vi "experiment control.vi"() -> ()   [LabVIEW 2012] (continued)
  out "dio64:debug2":T36(array[cluster])=[{"Begin (ms)"=0.0, "Duration (ms)"=0.1720000000000006, "DIO64 Line 1"=[FALSE, FALSE, FALSE, FALSE, FALSE, FALSE, FALSE, FALSE, FALSE, FALSE, FALSE, FALSE, FALSE, FALSE, FALSE, FALSE], "DIO64 Line 2"=[FALSE, FALSE, FALSE, FALSE, FALSE, FALSE, FALSE, FALSE, FALSE, FALSE, FALSE, FALSE, FALSE, FALSE, FALSE, FALSE], "DIO64 Line 3"=[FALSE, FALSE, FALSE, FALSE, FALSE, FALSE, FALSE, FALSE, FALSE, FALSE, FALSE, FALSE, FALSE, FALSE, FALSE, FALSE], "DIO64 Line 4"=[FALSE, FALSE, FALSE, FALSE, FALSE, FALSE, FALSE, FALSE, FALSE, FALSE, FALSE, FALSE, FALSE, FALSE, FALSE, FALSE]}, {"Begin (ms)"=0.1720000000000006, "Duration (ms)"=4.020009999999999, "DIO64 Line 1"=[FALSE, FALSE, FALSE, FALSE, FALSE, FALSE, FALSE, FALSE, FALSE, FALSE, FALSE, FALSE, FALSE, TRUE, FALSE, FALSE], "DIO64 Line 2"=[FALSE, FALSE, FALSE, FALSE, FALSE, FALSE, FALSE, FALSE, FALSE, FALSE, FALSE, FALSE, FALSE, FALSE, FALSE, TRUE], "DIO64 Line 3"=[FALSE, FALSE, FALSE, FALSE, FALSE, FALSE, FALSE, FALSE, FALSE, FALSE, FALSE, FALSE, FALSE, FALSE, FALSE, FALSE], "DIO64 Line 4"=[FALSE, FALSE, FALSE, FALSE, FALSE, FALSE, FALSE, FALSE, FALSE, FALSE, FALSE, FALSE, FALSE, FALSE, FALSE, FALSE]}, {"Begin (ms)"=4.19201, "Duration (ms)"=0.010000000000001563, "DIO64 Line 1"=[FALSE, FALSE, FALSE, FALSE, FALSE, FALSE, FALSE, FALSE, FALSE, FALSE, FALSE, FALSE, FALSE, TRUE, FALSE, FALSE], "DIO64 Line 2"=[FALSE, FALSE, FALSE, FALSE, FALSE, FALSE, FALSE, FALSE, FALSE, FALSE, FALSE, FALSE, FALSE, FALSE, FALSE, TRUE], "DIO64 Line 3"=[FALSE, FALSE, FALSE, FALSE, FALSE, FALSE, FALSE, FALSE, FALSE, FALSE, FALSE, FALSE, FALSE, FALSE, FALSE, FALSE], "DIO64 Line 4"=[FALSE, FALSE, FALSE, FALSE, FALSE, FALSE, FALSE, FALSE, FALSE, FALSE, FALSE, FALSE, FALSE, FALSE, FALSE, FALSE]}, {"Begin (ms)"=4.202010000000001, "Duration (ms)"=13.97239, "DIO64 Line 1"=[FALSE, FALSE, FALSE, FALSE, FALSE, FALSE, FALSE, FALSE, FALSE, FALSE, FALSE, FALSE, FALSE, TRUE, FALSE, FALSE], "DIO64 Line 2"=[FALSE, FALSE, FALSE, FALSE, FALSE, FALSE, FALSE, FALSE, FALSE, FALSE, FALSE, FALSE, FALSE, FALSE, FALSE, TRUE], "DIO64 Line 3"=[FALSE, FALSE, FALSE, FALSE, FALSE, FALSE, FALSE, FALSE, FALSE, FALSE, FALSE, FALSE, FALSE, FALSE, FALSE, FALSE], "DIO64 Line 4"=[FALSE, FALSE, FALSE, FALSE, FALSE, FALSE, FALSE, FALSE, FALSE, FALSE, FALSE, FALSE, FALSE, FALSE, FALSE, FALSE]}, {"Begin (ms)"=18.174400000000002, "Duration (ms)"=0.00999999999999801, "DIO64 Line 1"=[FALSE, FALSE, FALSE, FALSE, FALSE, FALSE, FALSE, FALSE, FALSE, FALSE, FALSE, FALSE, FALSE, TRUE, FALSE, FALSE], "DIO64 Line 2"=[FALSE, FALSE, FALSE, FALSE, FALSE, FALSE, FALSE, FALSE, FALSE, FALSE, FALSE, FALSE, FALSE, FALSE, FALSE, TRUE], "DIO64 Line 3"=[FALSE, FALSE, FALSE, FALSE, FALSE, FALSE, FALSE, FALSE, FALSE, FALSE, FALSE, FALSE, FALSE, FALSE, FALSE, FALSE], "DIO64 Line 4"=[TRUE, FALSE, FALSE, FALSE, FALSE, FALSE, FALSE, FALSE, FALSE, FALSE, FALSE, FALSE, FALSE, FALSE, FALSE, FALSE]}, {"Begin (ms)"=18.1844, "Duration (ms)"=0.9876000000000005, "DIO64 Line 1"=[FALSE, FALSE, FALSE, FALSE, FALSE, FALSE, FALSE, FALSE, FALSE, FALSE, FALSE, FALSE, FALSE, TRUE, FALSE, FALSE], "DIO64 Line 2"=[FALSE, FALSE, FALSE, FALSE, FALSE, FALSE, FALSE, FALSE, FALSE, FALSE, FALSE, FALSE, FALSE, FALSE, FALSE, TRUE], "DIO64 Line 3"=[FALSE, FALSE, FALSE, FALSE, FALSE, FALSE, FALSE, FALSE, FALSE, FALSE, FALSE, FALSE, FALSE, FALSE, FALSE, FALSE], "DIO64 Line 4"=[FALSE, FALSE, FALSE, FALSE, FALSE, FALSE, FALSE, FALSE, FALSE, FALSE, FALSE, FALSE, FALSE, FALSE, FALSE, FALSE]}, {"Begin (ms)"=19.172, "Duration (ms)"=0.010000000000001563, "DIO64 Line 1"=[FALSE, FALSE, FALSE, FALSE, FALSE, FALSE, FALSE, FALSE, FALSE, FALSE, FALSE, FALSE, FALSE, TRUE, FALSE, FALSE], "DIO64 Line 2"=[FALSE, FALSE, FALSE, FALSE, FALSE, FALSE, FALSE, FALSE, FALSE, TRUE, FALSE, FALSE, FALSE, FALSE, FALSE, TRUE], "DIO64 Line 3"=[FALSE, FALSE, FALSE, FALSE, FALSE, FALSE, FALSE, FALSE, FALSE, FALSE, FALSE, FALSE, FALSE, FALSE, FALSE, FALSE], "DIO64 Line 4"=[FALSE, FALSE, FALSE, FALSE, FALSE, FALSE, FALSE, FALSE, FALSE, FALSE, FALSE, FALSE, FALSE, FALSE, FALSE, FALSE]}, {"Begin (ms)"=19.182000000000002, "Duration (ms)"=0.136099999999999, "DIO64 Line 1"=[FALSE, FALSE, FALSE, FALSE, FALSE, FALSE, FALSE, FALSE, FALSE, FALSE, FALSE, FALSE, FALSE, TRUE, FALSE, FALSE], "DIO64 Line 2"=[FALSE, FALSE, FALSE, FALSE, FALSE, FALSE, FALSE, FALSE, FALSE, FALSE, FALSE, FALSE, FALSE, FALSE, FALSE, TRUE], "DIO64 Line 3"=[FALSE, FALSE, FALSE, FALSE, FALSE, FALSE, FALSE, FALSE, FALSE, FALSE, FALSE, FALSE, FALSE, FALSE, FALSE, FALSE], "DIO64 Line 4"=[FALSE, FALSE, FALSE, FALSE, FALSE, FALSE, FALSE, FALSE, FALSE, FALSE, FALSE, FALSE, FALSE, FALSE, FALSE, FALSE]}, {"Begin (ms)"=19.3181, "Duration (ms)"=0.010000000000001563, "DIO64 Line 1"=[FALSE, FALSE, FALSE, TRUE, FALSE, FALSE, FALSE, FALSE, FALSE, FALSE, FALSE, FALSE, FALSE, TRUE, TRUE, FALSE], "DIO64 Line 2"=[FALSE, FALSE, FALSE, FALSE, FALSE, FALSE, FALSE, FALSE, FALSE, FALSE, FALSE, FALSE, FALSE, FALSE, FALSE, TRUE], "DIO64 Line 3"=[FALSE, FALSE, FALSE, FALSE, FALSE, FALSE, FALSE, FALSE, FALSE, FALSE, FALSE, FALSE, FALSE, FALSE, FALSE, FALSE], "DIO64 Line 4"=[FALSE, FALSE, FALSE, FALSE, FALSE, FALSE, FALSE, FALSE, FALSE, FALSE, FALSE, FALSE, FALSE, FALSE, FALSE, FALSE]}, {"Begin (ms)"=19.328100000000003, "Duration (ms)"=0.054999999999999716, "DIO64 Line 1"=[FALSE, FALSE, FALSE, FALSE, FALSE, FALSE, FALSE, FALSE, FALSE, FALSE, FALSE, FALSE, FALSE, TRUE, TRUE, FALSE], "DIO64 Line 2"=[FALSE, FALSE, FALSE, FALSE, FALSE, FALSE, FALSE, FALSE, FALSE, FALSE, FALSE, FALSE, FALSE, FALSE, FALSE, TRUE], "DIO64 Line 3"=[FALSE, FALSE, FALSE, FALSE, FALSE, FALSE, FALSE, FALSE, FALSE, FALSE, FALSE, FALSE, FALSE, FALSE, FALSE, FALSE], "DIO64 Line 4"=[FALSE, FALSE, FALSE, FALSE, FALSE, FALSE, FALSE, FALSE, FALSE, FALSE, FALSE, FALSE, FALSE, FALSE, FALSE, FALSE]}, {"Begin (ms)"=19.383100000000002, "Duration (ms)"=0.06009999999999849, "DIO64 Line 1"=[FALSE, FALSE, FALSE, FALSE, FALSE, FALSE, FALSE, FALSE, FALSE, FALSE, FALSE, FALSE, FALSE, TRUE, FALSE, FALSE], "DIO64 Line 2"=[FALSE, FALSE, FALSE, FALSE, FALSE, FALSE, FALSE, FALSE, FALSE, FALSE, FALSE, FALSE, FALSE, FALSE, FALSE, TRUE], "DIO64 Line 3"=[FALSE, FALSE, FALSE, FALSE, FALSE, FALSE, FALSE, FALSE, FALSE, FALSE, FALSE, FALSE, FALSE, FALSE, FALSE, FALSE], "DIO64 Line 4"=[FALSE, FALSE, FALSE, FALSE, FALSE, FALSE, FALSE, FALSE, FALSE, FALSE, FALSE, FALSE, FALSE, FALSE, FALSE, FALSE]}, {"Begin (ms)"=19.4432, "Duration (ms)"=0.010000000000001563, "DIO64 Line 1"=[FALSE, FALSE, FALSE, FALSE, TRUE, FALSE, FALSE, FALSE, FALSE, FALSE, FALSE, FALSE, FALSE, TRUE, FALSE, FALSE], "DIO64 Line 2"=[FALSE, FALSE, FALSE, FALSE, FALSE, FALSE, FALSE, FALSE, FALSE, FALSE, FALSE, FALSE, FALSE, FALSE, FALSE, TRUE], "DIO64 Line 3"=[FALSE, FALSE, FALSE, FALSE, FALSE, FALSE, FALSE, FALSE, FALSE, FALSE, FALSE, FALSE, FALSE, FALSE, FALSE, FALSE], "DIO64 Line 4"=[FALSE, FALSE, FALSE, FALSE, FALSE, FALSE, FALSE, FALSE, FALSE, FALSE, FALSE, FALSE, FALSE, FALSE, FALSE, FALSE]}, {"Begin (ms)"=19.453200000000002, "Duration (ms)"=0.6777999999999977, "DIO64 Line 1"=[FALSE, FALSE, FALSE, FALSE, FALSE, FALSE, FALSE, FALSE, FALSE, FALSE, FALSE, FALSE, FALSE, TRUE, FALSE, FALSE], "DIO64 Line 2"=[FALSE, FALSE, FALSE, FALSE, FALSE, FALSE, FALSE, FALSE, FALSE, FALSE, FALSE, FALSE, FALSE, FALSE, FALSE, TRUE], "DIO64 Line 3"=[FALSE, FALSE, FALSE, FALSE, FALSE, FALSE, FALSE, FALSE, FALSE, FALSE, FALSE, FALSE, FALSE, FALSE, FALSE, FALSE], "DIO64 Line 4"=[FALSE, FALSE, FALSE, FALSE, FALSE, FALSE, FALSE, FALSE, FALSE, FALSE, FALSE, FALSE, FALSE, FALSE, FALSE, FALSE]}, {"Begin (ms)"=20.131, "Duration (ms)"=0.03999999999999915, "DIO64 Line 1"=[FALSE, FALSE, FALSE, FALSE, FALSE, FALSE, FALSE, FALSE, FALSE, TRUE, TRUE, FALSE, FALSE, TRUE, FALSE, FALSE], "DIO64 Line 2"=[FALSE, FALSE, FALSE, FALSE, FALSE, FALSE, FALSE, FALSE, FALSE, FALSE, FALSE, FALSE, FALSE, FALSE, FALSE, TRUE], "DIO64 Line 3"=[FALSE, FALSE, FALSE, FALSE, FALSE, FALSE, FALSE, FALSE, FALSE, FALSE, FALSE, FALSE, FALSE, FALSE, FALSE, FALSE], "DIO64 Line 4"=[FALSE, FALSE, FALSE, FALSE, FALSE, FALSE, FALSE, FALSE, FALSE, FALSE, FALSE, FALSE, FALSE, FALSE, FALSE, FALSE]}, {"Begin (ms)"=20.171, "Duration (ms)"=0.0010000000000012221, "DIO64 Line 1"=[FALSE, FALSE, FALSE, FALSE, FALSE, FALSE, FALSE, FALSE, FALSE, TRUE, FALSE, FALSE, FALSE, TRUE, FALSE, FALSE], "DIO64 Line 2"=[FALSE, FALSE, FALSE, FALSE, FALSE, FALSE, FALSE, FALSE, FALSE, FALSE, FALSE, FALSE, FALSE, FALSE, FALSE, TRUE], "DIO64 Line 3"=[FALSE, FALSE, FALSE, FALSE, FALSE, FALSE, FALSE, FALSE, FALSE, FALSE, FALSE, FALSE, FALSE, FALSE, FALSE, FALSE], "DIO64 Line 4"=[FALSE, FALSE, FALSE, FALSE, FALSE, FALSE, FALSE, FALSE, FALSE, FALSE, FALSE, FALSE, FALSE, FALSE, FALSE, FALSE]}, {"Begin (ms)"=20.172, "Duration (ms)"=2.0, "DIO64 Line 1"=[FALSE, FALSE, FALSE, FALSE, FALSE, FALSE, TRUE, FALSE, FALSE, FALSE, FALSE, FALSE, FALSE, TRUE, FALSE, FALSE], "DIO64 Line 2"=[FALSE, FALSE, FALSE, FALSE, TRUE, FALSE, FALSE, FALSE, FALSE, FALSE, FALSE, FALSE, FALSE, TRUE, FALSE, TRUE], "DIO64 Line 3"=[FALSE, FALSE, FALSE, TRUE, FALSE, FALSE, FALSE, FALSE, FALSE, FALSE, FALSE, FALSE, FALSE, FALSE, FALSE, FALSE], "DIO64 Line 4"=[FALSE, FALSE, FALSE, FALSE, FALSE, FALSE, FALSE, FALSE, FALSE, FALSE, FALSE, FALSE, FALSE, FALSE, FALSE, TRUE]}, {"Begin (ms)"=22.172, "Duration (ms)"=0.004999999999999005, "DIO64 Line 1"=[FALSE, FALSE, FALSE, FALSE, FALSE, FALSE, FALSE, FALSE, FALSE, TRUE, FALSE, FALSE, FALSE, TRUE, FALSE, FALSE], "DIO64 Line 2"=[FALSE, FALSE, FALSE, FALSE, FALSE, FALSE, FALSE, FALSE, FALSE, FALSE, FALSE, TRUE, FALSE, FALSE, FALSE, TRUE], "DIO64 Line 3"=[FALSE, FALSE, FALSE, FALSE, FALSE, FALSE, FALSE, FALSE, FALSE, FALSE, FALSE, FALSE, FALSE, FALSE, FALSE, FALSE], "DIO64 Line 4"=[FALSE, FALSE, FALSE, FALSE, FALSE, FALSE, FALSE, FALSE, FALSE, FALSE, FALSE, FALSE, FALSE, FALSE, FALSE, FALSE]}, {"Begin (ms)"=22.177, "Duration (ms)"=0.005000000000002558, "DIO64 Line 1"=[FALSE, FALSE, FALSE, FALSE, FALSE, FALSE, FALSE, FALSE, FALSE, TRUE, TRUE, FALSE, FALSE, TRUE, FALSE, FALSE], "DIO64 Line 2"=[FALSE, FALSE, FALSE, FALSE, FALSE, FALSE, FALSE, FALSE, FALSE, FALSE, FALSE, TRUE, FALSE, FALSE, FALSE, TRUE], "DIO64 Line 3"=[FALSE, FALSE, FALSE, FALSE, FALSE, FALSE, FALSE, FALSE, FALSE, FALSE, FALSE, FALSE, FALSE, FALSE, FALSE, FALSE], "DIO64 Line 4"=[FALSE, FALSE, FALSE, FALSE, FALSE, FALSE, FALSE, FALSE, FALSE, FALSE, FALSE, FALSE, FALSE, FALSE, FALSE, FALSE]}, {"Begin (ms)"=22.182000000000002, "Duration (ms)"=0.004999999999999005, "DIO64 Line 1"=[FALSE, FALSE, FALSE, FALSE, FALSE, FALSE, FALSE, FALSE, FALSE, TRUE, TRUE, FALSE, FALSE, TRUE, FALSE, FALSE], "DIO64 Line 2"=[FALSE, FALSE, FALSE, FALSE, FALSE, FALSE, FALSE, FALSE, FALSE, FALSE, FALSE, FALSE, FALSE, FALSE, FALSE, TRUE], "DIO64 Line 3"=[FALSE, FALSE, FALSE, FALSE, FALSE, FALSE, FALSE, FALSE, FALSE, FALSE, FALSE, FALSE, FALSE, FALSE, FALSE, FALSE], "DIO64 Line 4"=[FALSE, FALSE, FALSE, FALSE, FALSE, FALSE, FALSE, FALSE, FALSE, FALSE, FALSE, FALSE, FALSE, FALSE, FALSE, FALSE]}, {"Begin (ms)"=22.187, "Duration (ms)"=0.005009999999998627, "DIO64 Line 1"=[FALSE, FALSE, FALSE, FALSE, FALSE, FALSE, FALSE, TRUE, FALSE, TRUE, TRUE, FALSE, FALSE, TRUE, FALSE, FALSE], "DIO64 Line 2"=[FALSE, FALSE, FALSE, FALSE, FALSE, FALSE, FALSE, FALSE, FALSE, FALSE, FALSE, FALSE, FALSE, FALSE, FALSE, TRUE], "DIO64 Line 3"=[FALSE, FALSE, FALSE, FALSE, FALSE, FALSE, FALSE, FALSE, FALSE, FALSE, FALSE, FALSE, FALSE, FALSE, FALSE, FALSE], "DIO64 Line 4"=[FALSE, TRUE, FALSE, FALSE, FALSE, FALSE, FALSE, FALSE, FALSE, FALSE, FALSE, FALSE, FALSE, FALSE, FALSE, FALSE]}, {"Begin (ms)"=22.19201, "Duration (ms)"=0.004989999999999384, "DIO64 Line 1"=[FALSE, FALSE, FALSE, FALSE, FALSE, FALSE, FALSE, TRUE, FALSE, TRUE, TRUE, FALSE, FALSE, TRUE, FALSE, FALSE], "DIO64 Line 2"=[FALSE, FALSE, FALSE, FALSE, FALSE, FALSE, FALSE, FALSE, FALSE, FALSE, FALSE, FALSE, FALSE, FALSE, FALSE, TRUE], "DIO64 Line 3"=[FALSE, FALSE, FALSE, FALSE, FALSE, FALSE, FALSE, FALSE, FALSE, FALSE, FALSE, FALSE, FALSE, FALSE, FALSE, FALSE], "DIO64 Line 4"=[FALSE, TRUE, FALSE, FALSE, FALSE, FALSE, FALSE, FALSE, FALSE, FALSE, FALSE, FALSE, FALSE, FALSE, FALSE, FALSE]}, {"Begin (ms)"=22.197, "Duration (ms)"=0.005010000000002179, "DIO64 Line 1"=[FALSE, FALSE, FALSE, FALSE, FALSE, FALSE, FALSE, FALSE, FALSE, TRUE, TRUE, FALSE, FALSE, TRUE, FALSE, FALSE], "DIO64 Line 2"=[FALSE, FALSE, FALSE, FALSE, FALSE, FALSE, FALSE, FALSE, FALSE, FALSE, FALSE, FALSE, FALSE, FALSE, FALSE, TRUE], "DIO64 Line 3"=[FALSE, FALSE, FALSE, FALSE, FALSE, FALSE, FALSE, FALSE, FALSE, FALSE, FALSE, FALSE, FALSE, FALSE, FALSE, FALSE], "DIO64 Line 4"=[FALSE, FALSE, FALSE, FALSE, FALSE, FALSE, FALSE, FALSE, FALSE, FALSE, FALSE, FALSE, FALSE, FALSE, FALSE, FALSE]}, {"Begin (ms)"=22.20201, "Duration (ms)"=9.974989999999998, "DIO64 Line 1"=[FALSE, FALSE, FALSE, FALSE, FALSE, FALSE, FALSE, FALSE, FALSE, TRUE, TRUE, FALSE, FALSE, TRUE, FALSE, FALSE], "DIO64 Line 2"=[FALSE, FALSE, FALSE, FALSE, FALSE, FALSE, FALSE, FALSE, FALSE, FALSE, FALSE, FALSE, FALSE, FALSE, FALSE, TRUE], "DIO64 Line 3"=[FALSE, FALSE, FALSE, FALSE, FALSE, FALSE, FALSE, FALSE, FALSE, FALSE, FALSE, FALSE, FALSE, FALSE, FALSE, FALSE], "DIO64 Line 4"=[FALSE, FALSE, FALSE, FALSE, FALSE, FALSE, FALSE, FALSE, FALSE, FALSE, FALSE, FALSE, FALSE, FALSE, FALSE, FALSE]}, {"Begin (ms)"=32.177, "Duration (ms)"=67.995, "DIO64 Line 1"=[FALSE, FALSE, FALSE, FALSE, FALSE, FALSE, FALSE, FALSE, FALSE, FALSE, FALSE, FALSE, FALSE, TRUE, FALSE, FALSE], "DIO64 Line 2"=[FALSE, FALSE, FALSE, FALSE, FALSE, FALSE, FALSE, FALSE, FALSE, FALSE, FALSE, FALSE, FALSE, FALSE, FALSE, TRUE], "DIO64 Line 3"=[FALSE, FALSE, FALSE, FALSE, FALSE, FALSE, FALSE, FALSE, FALSE, FALSE, FALSE, FALSE, FALSE, FALSE, FALSE, FALSE], "DIO64 Line 4"=[FALSE, FALSE, FALSE, FALSE, FALSE, FALSE, FALSE, FALSE, FALSE, FALSE, FALSE, FALSE, FALSE, FALSE, FALSE, FALSE]}, {"Begin (ms)"=100.172, "Duration (ms)"=99.828, "DIO64 Line 1"=[FALSE, FALSE, FALSE, FALSE, FALSE, FALSE, FALSE, FALSE, FALSE, FALSE, FALSE, FALSE, FALSE, FALSE, FALSE, FALSE], "DIO64 Line 2"=[FALSE, FALSE, FALSE, FALSE, FALSE, FALSE, FALSE, FALSE, FALSE, FALSE, FALSE, FALSE, FALSE, FALSE, FALSE, FALSE], "DIO64 Line 3"=[FALSE, FALSE, FALSE, FALSE, FALSE, FALSE, FALSE, FALSE, FALSE, FALSE, FALSE, FALSE, FALSE, FALSE, FALSE, FALSE], "DIO64 Line 4"=[FALSE, FALSE, FALSE, FALSE, FALSE, FALSE, FALSE, FALSE, FALSE, FALSE, FALSE, FALSE, FALSE, FALSE, FALSE, FALSE]}] caption="DIO64 Debug Timing"
  out "dio64:debug1":T37(array[cluster])=[{"Task"="T0", "begin time"=0.0, "end time"=0.0, "Chops"=[]}, {"Task"="Bertha UV Shutter", "begin time"=0.1720000000000006, "end time"=100.172, "Chops"=[FALSE, FALSE, FALSE, FALSE, FALSE, FALSE, FALSE, FALSE, FALSE, FALSE, FALSE, FALSE]}, {"Task"="Jessica Shutter", "begin time"=0.1720000000000006, "end time"=100.172, "Chops"=[FALSE, FALSE, FALSE, FALSE, FALSE, FALSE, FALSE, FALSE, FALSE, FALSE, FALSE, FALSE]}, {"Task"="Framegrabber Trigger", "begin time"=4.19201, "end time"=4.202010000000001, "Chops"=[TRUE, TRUE, TRUE, TRUE, TRUE, TRUE, FALSE, FALSE, FALSE, FALSE, FALSE, FALSE]}, {"Task"="IOUpdate", "begin time"=18.174400000000002, "end time"=18.1844, "Chops"=[FALSE, FALSE, FALSE, FALSE, FALSE, FALSE, FALSE, FALSE, FALSE, FALSE, FALSE, FALSE]}, {"Task"="Trigger DAC", "begin time"=19.172, "end time"=19.182000000000002, "Chops"=[FALSE, FALSE, FALSE, FALSE, FALSE, FALSE, FALSE, FALSE, FALSE, FALSE, FALSE, FALSE]}, {"Task"="Abby Flashlamp", "begin time"=19.3181, "end time"=19.328100000000003, "Chops"=[FALSE, FALSE, FALSE, FALSE, FALSE, FALSE, FALSE, FALSE, FALSE, FALSE, FALSE, FALSE]}, {"Task"="Gas Pulse", "begin time"=19.3181, "end time"=19.383100000000002, "Chops"=[FALSE, FALSE, FALSE, FALSE, FALSE, FALSE, FALSE, FALSE, FALSE, FALSE, FALSE, FALSE]}, {"Task"="Abby Q-switch", "begin time"=19.4432, "end time"=19.453200000000002, "Chops"=[FALSE, FALSE, FALSE, FALSE, FALSE, FALSE, FALSE, FALSE, FALSE, FALSE, FALSE, FALSE]}, {"Task"="Zero DAC", "begin time"=20.131, "end time"=20.171, "Chops"=[FALSE, FALSE, FALSE, FALSE, FALSE, FALSE, FALSE, FALSE, FALSE, FALSE, FALSE, FALSE]}, {"Task"="Stop Ions", "begin time"=20.171, "end time"=20.172, "Chops"=[FALSE, FALSE, FALSE, FALSE, FALSE, FALSE, FALSE, FALSE, FALSE, FALSE, FALSE, FALSE]}, {"Task"="Trap", "begin time"=20.172, "end time"=22.172, "Chops"=[FALSE, FALSE, FALSE, FALSE, FALSE, FALSE, FALSE, FALSE, FALSE, FALSE, FALSE, FALSE]}, {"Task"="Kick to MCP", "begin time"=22.172, "end time"=22.177, "Chops"=[FALSE, FALSE, FALSE, FALSE, FALSE, FALSE, FALSE, FALSE, FALSE, FALSE, FALSE, FALSE]}, {"Task"="Scope trigger 2", "begin time"=22.172, "end time"=22.182000000000002, "Chops"=[TRUE, TRUE, TRUE, FALSE, FALSE, FALSE, FALSE, FALSE, FALSE, FALSE, FALSE, FALSE]}, {"Task"="Zero DAC", "begin time"=22.177, "end time"=32.177, "Chops"=[FALSE, FALSE, FALSE, FALSE, FALSE, FALSE, FALSE, FALSE, FALSE, FALSE, FALSE, FALSE]}, {"Task"="Trigger Scope", "begin time"=22.187, "end time"=22.197, "Chops"=[FALSE, FALSE, FALSE, FALSE, FALSE, FALSE, TRUE, FALSE, FALSE, FALSE, FALSE, FALSE]}, {"Task"="Img MCP Trigger", "begin time"=22.19201, "end time"=22.20201, "Chops"=[TRUE, TRUE, TRUE, TRUE, TRUE, TRUE, FALSE, FALSE, FALSE, FALSE, FALSE, FALSE]}] caption="DIO64 Debug Timing" {"end time" format="%#_8g"; "begin time" format="%#_8g"}
  out "toptica:task:skip":refnum<k21>
  out "stella:task:skip":refnum<k21>
  out "TDS5034B Data":cluster{"Y":dbl[], "t0":dbl, "dt":dbl}[](array[cluster])=[{"Y"=array[2500 elements], "t0"=3.7485e-09, "dt"=4e-09}]
  out "documentation":string[](array[string])=["Initialize the shift-register data, here.\n(data names are defined by what you wire into the bundle function)", "Cleanup any data and references, here.\n(this is called automatically, by the Macro: Exit)", "Initialize the User Interface, here.\n(this is called automatically, by the Macro: Init)", "Set and Unset Cursor Busy.\n(Usage: \"UI: Cursor Set >> Busy|Idle\")", "Argument", "Gets the program states from the main loop case selector\n(Usage: \"UI: Get Case Strings\")", "Gets program documentation from main loop case selector\n(Usage: \"UI: Get Case Documentation\")", "Updates DIO64 control with string from DIO64 Tasks\n(Usage: \"call after any modification to DIO64 Tasks\")", "Updates DIO64 control with string from DIO64 Tasks\n(Usage: \"call after any modification to DIO64 Tasks\")", "Updates DIO64 control with string from DIO64 Tasks\n(Usage: \"call after any modification to DIO64 Tasks\")", "Initialization Macro\n(This is called once, when the VI starts. It calls a number of other program states.)", "Exit Macro\n(This is called once, when the VI exits)", "Delays for some number of milliseconds\n(Usage: delay >>  TIME)", "Prints a message to the labview stdout control\n(Usage: stdout >> TEXT)", "Clears the queue\n(Usage: abort)", "Runs the test sequence\n(Usage: Test)", "Pauses the state machine\n(swaps out the queue to memory)", "Pauses the state machine\n(swaps out the queue to memory)", "Pauses the state machine\n(swaps out the queue to memory)", "Pauses the state machine\n(swaps out the queue to memory)", "Initialize the DIO64", "Parses the DIO64\n(Usage: DIO64: Prepare >> CHOP)", "Updates the DIO64 Timing Graph\n(Usage: call whenever the DIO64 changes)", "Runs the DIO64\n(Usage: DIO64: Run )\n(Usage: DIO64: Run >> Chop,CHOP to run CHOP a number of times in the frame control)\n(Usage: DIO64: Run >> Repeat,N, to run the prepared sequence N times)", "DIO64: Override\n(Usage: DIO64: Override >> CHANNEL, to run a channel like A0 or C6)", "Closes the DIO64\n(Usage: DIO64: Close)", "Initalize the Scope\n(Usage: Scope: Initialize >> SCOPE, where SCOPE can be DPO)", "Updates Scope Settings\n(Usage: Scope: Settings >> SCOPE, where SCOPE can be DPO)", "Reads a frame from the Scope\n(Usage: Scope: Read >> SCOPE, where SCOPE can be DPO)", "Close the Scope\n(Usage: Scope: Close >> SCOPE, where SCOPE can be DPO)"] caption="Documentation"
  in  "Coils AO Task:skip":refnum<k21>
  in  "Coils DO Task:skip":refnum<k21>
  out "Waveform Chart":waveform(dbl)[](graph)=[{"t0"=timestamp(0 s since 1904-01-01), "dt"=4e-09, "Y"=array[2500 elements]}]
  in  "stdin":string="Magnetometer: Close"
  # "Task Name"
  # "Start (ms)"
  # "Edge"
  # "Reference"
  # "End (ms)"
  # "Edge"
  # "Reference"
  # "Time (ms)"
  # "A0"
  # "A1"
  # "A2"
  # "A3"
  # "A4"
  # "A5"
  # "A6"
  # "Time (ms)"
  # "A0"
  # "A1"
  # "A2"
  # "A3"
  # "A4"
  # "A5"
  # "A6"
  # "A7"
  # "0"
  # "1"
  # "2"
  # "3"
  # "4"
  # "5"
  # "6"
  # "7"
  # "8"
  # "9"
  # "10"
  # "11"
  # "AO1"
  # "DO1 - Abby intlk 1"
  # "DI1"
  # "DO2 - Abby intlk 2"
  # "DI2"
  # "AO2"
  # "DO3 - Bertha WP flip"
  # "DI3"
  # "AI1"
  # "DO4 - Depletion flip"
  # "DI4"
  # "AI2"
  # "DO5"
  # "DI5"
  # "DO6"
  # "DO7"
  # "DO8"
  # "V"
  # "kHz"
  # "mVpp"
  # "deg"
  # "Freq (Hz)"
  # "Phase (deg)"
  # "Duty Cyc. (%)"
  # "Trig."
  # "1"
  # "2"
  # "(A)"
  # "(A)"
  # "(A)"
  # "(V)"
  # "(A)"
  # "(A)"
  # "(A)"
  # "(V)"
  # "(A)"
  # "(A)"
  # "(A)"
  # "(V)"
  # "(A)"
  # "(A)"
  # "(A)"
  # "(V)"
  # "nm"
  # "cm-1"
  # "Stella"
  # "Toptica"
  # "Frequency (kHz)"
  # "Phase"
  # "Amplitude"
  # "1"
  # "2"
  # "3"
  # "4"
  # "5"
  # "6"
  # "x 20 us"
  # "For Profile Pin\nAmplitude Ramps"
  # "Start"
  # "End"
  # "Ramp Time (us)"
  # "R0"
  # "R1"
  # "R2"
  # "R3"
  # "R4"
  # "R5"
  # "R6"
  # "R7"
  # "R8"
  # "R9"
  # "Hz"
  # "Hz"
  # "Hz"
  # "V"
  # "V"
  # "V"
  # "V"
  # "0"
  # "1"
  # "2"
  # "3"
  # "0"
  # "1"
  # "2"
  # "3"
  # "4"
  # "5"
  # "6"
  # "7"
  # "8"
  # "9"
  # "10"
  # "A00"
  # "A01"
  # "A02"
  # "A03"
  # "A04"
  # "A05"
  # "A06"
  # "A07"
  # "A08"
  # "A09"
  # "A10"
  # "A11"
  # "A12"
  # "A13"
  # "A14"
  # "A15"
  # "B00"
  # "B01"
  # "B02"
  # "B03"
  # "B04"
  # "B05"
  # "B06"
  # "B07"
  # "B08"
  # "B09"
  # "B10"
  # "B11"
  # "B12"
  # "B13"
  # "B14"
  # "B15"
  # "C00"
  # "C01"
  # "C02"
  # "C03"
  # "C04"
  # "C05"
  # "C06"
  # "C07"
  # "C08"
  # "C09"
  # "C10"
  # "C11"
  # "C12"
  # "C13"
  # "C14"
  # "C15"
  # "D00"
  # "D01"
  # "D02"
  # "D03"
  # "D04"
  # "D05"
  # "D06"
  # "D07"
  # "D08"
  # "D09"
  # "D10"
  # "D11"
  # "D12"
  # "D13"
  # "D14"
  # "D15"
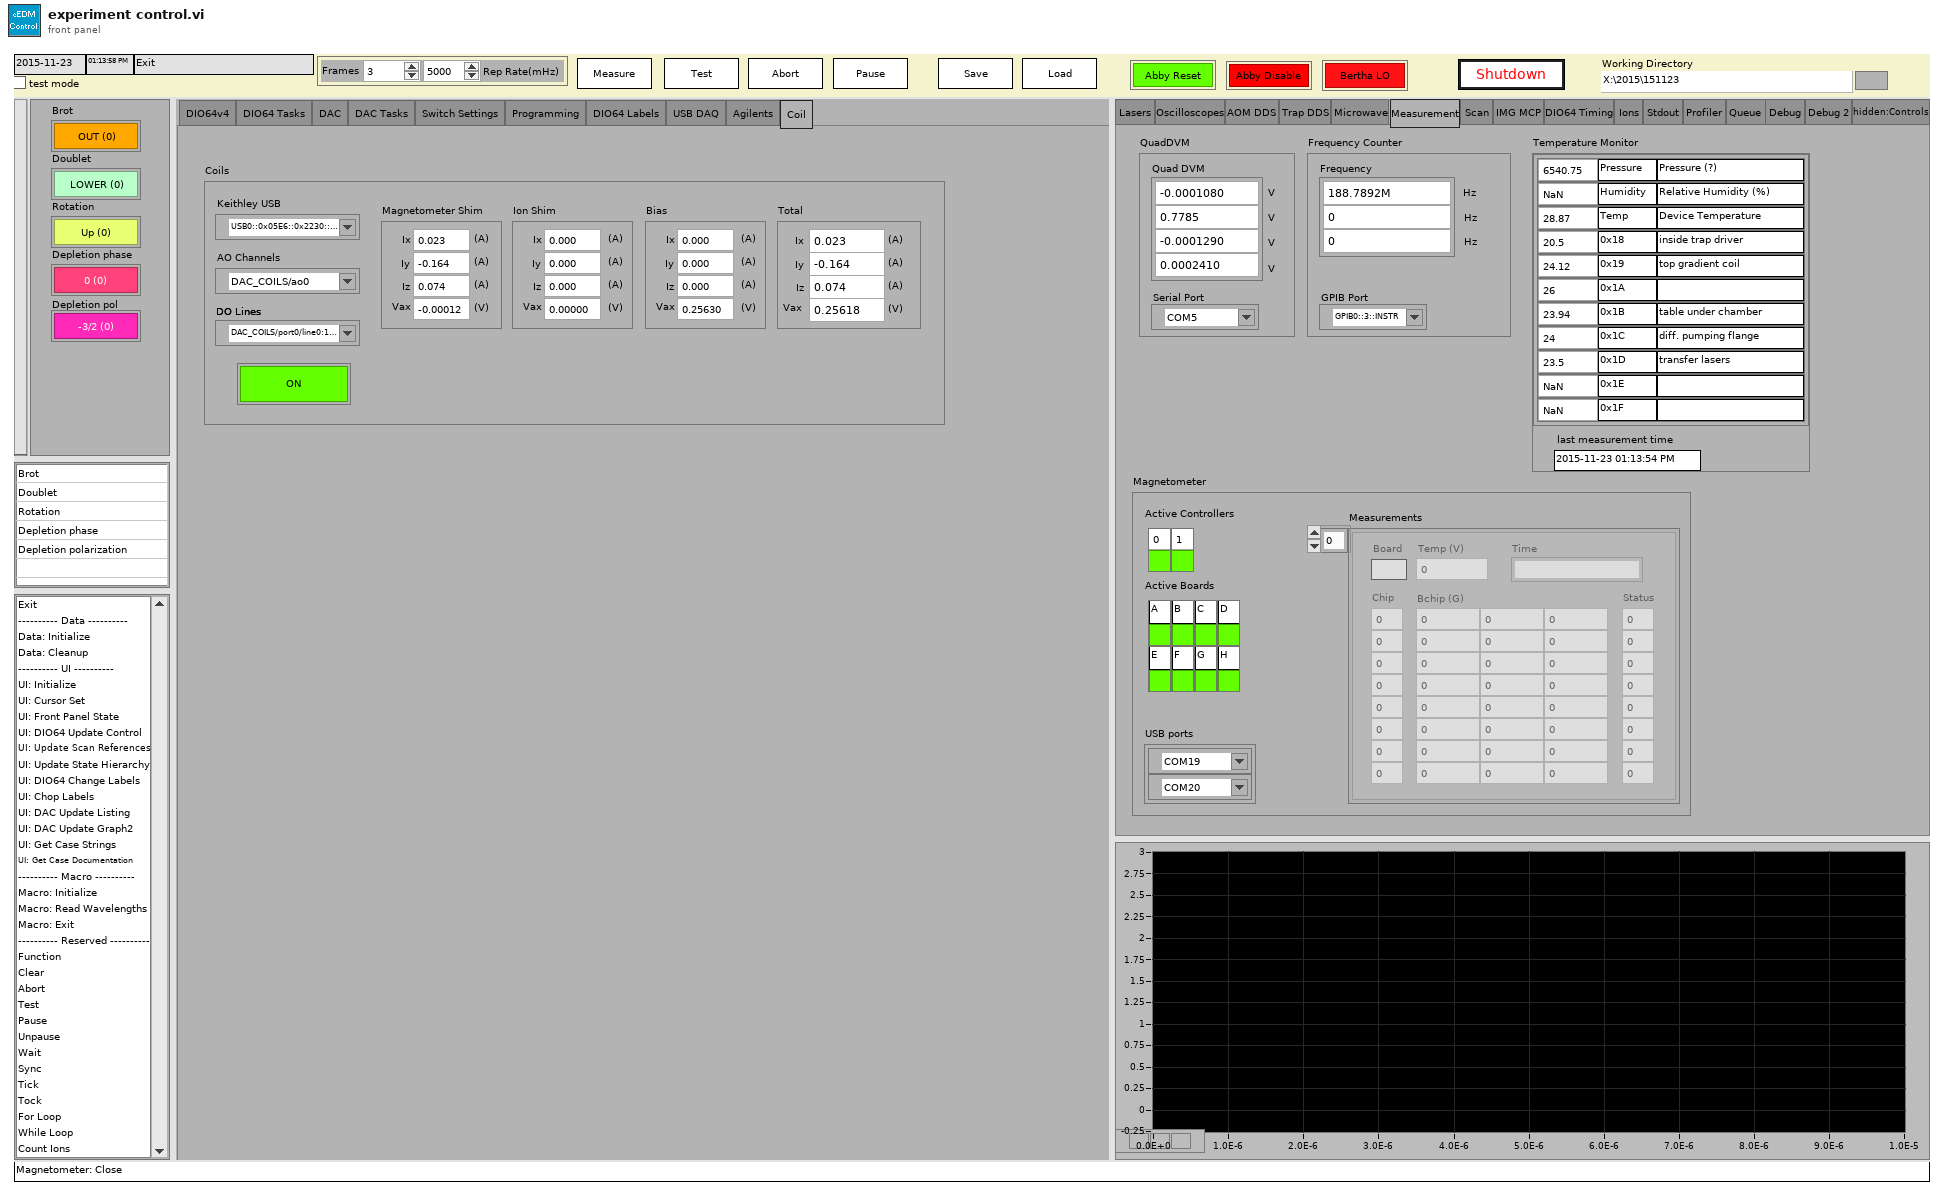
[diagram p1: front panel]
types:
  T1 = cluster{"Brot":bool, "Doublet":bool, "Rotation":bool, "Depletion phase":bool, "Depletion pol":bool}
  T2 = enum32{"DIO64v4", "DIO64 Tasks", "DAC", "DAC Tasks", "Switch Settings", "Programming", "DIO64 Labels", "USB DAQ", "Agilents", "Coil"}
  T3 = cluster{"Task":string, "begin time":dbl, "begin edge":bool, "begin reference":string, "end time":dbl, "end edge":bool, "end reference":string, "Chops":bool[]}[]
  T4 = cluster{"Name":string, "DIO64 Line 1":bool[], "DIO64 Line 2":bool[], "DIO64 Line 3":bool[], "DIO64 Line 4":bool[]}[]
  T5 = cluster{"Channel 1":picture[], "Channel 2":picture[], "Channel 3":picture[], "Channel 4":picture[]}
  T6 = cluster{"Task":string, "Reference":string, "Begin":dbl, "Chops 2":bool[]}[]
  T7 = cluster{"loaded":bool, "output 1":refnum<k21>, "clock 1":refnum<k21>, "output 2":refnum<k21>, "clock 2":refnum<k21>}
  T8 = cluster{"Name":string, "DAC":cluster{"Time":dbl, "Voltage":dbl[]}[]}[]
  T9 = cluster{"Brot":cluster{"in":dbl, "out":dbl}, "Doublet":cluster{"upper":dbl, "lower":dbl, "DurationUpper":dbl, "DurationLower":dbl, "Upper T":dbl, "Lower T":dbl}, "Rotation":cluster{"Down":cluster{"Frequency":dbl, "Phase":dbl, "Amplitude":dbl}[], "Up":cluster{"Frequency":dbl, "Phase":dbl, "Amplitude":dbl}[]}, "Depletion phase":cluster{"0 phase":dbl, "pi phase":dbl}}
  T10 = cluster{"Channel":string, "Name":string, "plot":bool}[][]
  T11 = cluster{"Digital Out":bool[], "Digital In":bool[], "Analog Out":u8[], "Analog In":u8[]}
  T12 = cluster{"Chillax":refnum<visa-resource-name>, "Output":bool, "Chillax Voltage":dbl, "Unchillax":refnum<visa-resource-name>}
  T13 = cluster{"USB":refnum<visa-resource-name>, "Amplitude":dbl, "Frequency":dbl, "Phase":dbl, "Upload":bool, "Output":bool}
  T14 = cluster{"USB":refnum<visa-resource-name>, "Upload":bool, "Output":bool, "Channels":cluster{"Frequency":dbl, "Phase":dbl, "Duty Cycle":dbl, "Trigger":bool}[], "Output Select":bool, "Amplitude":dbl, "Offset":dbl}
  T15 = cluster{"AO Channels":tag, "DO Lines":tag, "Keithley USB":refnum<visa-resource-name>, "Current Toggle":bool, "Magnetometer Shim":cluster{"x":dbl, "y":dbl, "z":dbl, "axgrad":dbl}, "Ion Shim":cluster{"x":dbl, "y":dbl, "z":dbl, "axgrad":dbl}, "Bias":cluster{"x":dbl, "y":dbl, "z":dbl, "axgrad":dbl}, "Total":cluster{"x":dbl, "y":dbl, "z":dbl, "axgrad":dbl}}
  T16 = enum32{"Lasers", "Oscilloscopes", "AOM DDS", "Trap DDS", "Microwave", "Measurement", "Scan", "IMG MCP", "DIO64 Timing", "Ions", "Stdout", "Profiler", "Queue", "Debug", "Debug 2", "hidden:Controls"}
  T17 = typedef "Laser.ctl" = cluster{"wavelength":dbl, "locked":bool, "lock tolerance":dbl, "setpoint":dbl, "scan start":dbl, "scan end":dbl, "progress":u8, "scan step":dbl, "scan":bool, "wavelengths":dbl[]}
  T18 = cluster{"wavelength":dbl, "scan start":dbl, "scan end":dbl, "progress":u8, "scan step":dbl, "scan":bool, "setpoint":dbl, "wavelengths":dbl[], "Channel":tag, "wavelength 2":dbl}
  T19 = cluster{"wavelength":dbl, "locked":bool, "scan start":dbl, "scan end":dbl, "progress":u8, "scan step":dbl, "scan":bool, "AI Channel":tag}
  T20 = cluster{"wavelength":dbl, "locked":bool, "lock tolerance":dbl, "setpoint":dbl, "scan start":dbl, "scan end":dbl, "progress":u8, "scan step":dbl, "scan":bool, "AI Channel":tag}
  T21 = cluster{"wavelength":dbl, "locked":bool, "DIO64":string, "scan start":dbl, "scan end":dbl, "progress":u8, "scan step":dbl, "scan":bool, "setpoint":dbl}
  T22 = cluster{"wavelength":dbl, "locked":bool, "DIO64":string, "scan start":dbl, "scan end":dbl, "progress":u8, "scan step":dbl, "scan":bool, "setpoint":dbl, "wavelengths":dbl[]}
  T23 = cluster{"Serial Port":refnum<visa-resource-name>, "Wavelength":dbl, "Units":string, "VISA Name":refnum<visa-resource-name>, "Reading":bool, "Detected":bool}
  T24 = cluster{"GPIB Address":refnum<visa-resource-name>, "Detected":bool, "Channels":u16[], "Resolution":u16, "Frames":u16, "Trigger Position":dbl, "Trigger Level":dbl, "Measurements":cluster{"Type":string, "Value":dbl, "Source":string}[]}
  T25 = cluster{"address":refnum<visa-resource-name>, "channel 1":dbl, "channel 2":dbl, "channel 3":dbl, "channel 4":dbl, "clock":dbl, "pll multiplier":u8, "vco gain":bool, "detected":bool, "channel 1 endramp":dbl, "channel 2 endramp":dbl, "channel 3 endramp":dbl, "channel 4 endramp":dbl, "frequency ramp":bool}
  T26 = cluster{"channels":cluster{"Frequency":dbl, "Phase":dbl, "Amplitude":dbl}[], "usb 1":refnum<visa-resource-name>, "usb 2":refnum<visa-resource-name>, "clock":dbl, "pll multiplier":u8, "ioupdate":bool, "detected":bool, "ramp":cluster{"start":dbl, "end":dbl, "ramp time":u8, "edge":bool}[], "232":refnum<visa-resource-name>, "load ARR":bool, "ramp enable":bool, "ramp time":u8, "Global\nScale Factor":dbl}
  T27 = cluster{"GPIB Port":refnum<visa-resource-name>, "detected":bool, "rf":bool, "frequency":dbl, "stop frequency":dbl, "power":dbl, "sweep time":dbl, "Chirp":bool, "Pulse Modulate":bool, "Set frequency":dbl}
  T28 = cluster{"Active Boards":cluster{"Status":bool, "Board":string}[][], "USB ports":refnum<visa-resource-name>[], "Active Controllers":cluster{"Status":bool, "Number":dbl}[], "Measurements":cluster{"Bchip":dbl[][], "Status":dbl[], "Temperature":dbl, "Chip":dbl[], "Board":string, "Time":string}[]}
  T29 = cluster{"measurements":cluster{"measurement":dbl, "location":string, "label":string}[], "last measurement time":string}
  T30 = cluster{"GPIB Port":refnum<visa-resource-name>, "Frequency":dbl[]}
  T31 = cluster{"Serial Port":refnum<visa-resource-name>, "Quad DVM":dbl[][]}
  T32 = cluster{"variable":string, "scan string":string, "randomize":bool, "enable":bool}[]
  T33 = cluster{"scan":bool, "Reference":string, "equation":string, "index":i32, "progress":u8, "next":dbl}[]
  T34 = cluster{"Hf  time threshold":dbl, "Ion Calibration":dbl, "Hf integrated":dbl, "HfF":dbl, "Hf integrated history":dbl[], "HfF history":dbl[], "<Hf integrated>":dbl, "<HfF>":dbl, "XY Graph":cluster{dbl, dbl}[], "History":u32, "Clear History":bool}
  T35 = cluster{"DIO64 Line 1":bool[], "DIO64 Line 2":bool[], "DIO64 Line 3":bool[], "DIO64 Line 4":bool[]}
  T36 = cluster{"Begin (ms)":dbl, "Duration (ms)":dbl, "DIO64 Line 1":bool[], "DIO64 Line 2":bool[], "DIO64 Line 3":bool[], "DIO64 Line 4":bool[]}[]
  T37 = cluster{"Task":string, "begin time":dbl, "end time":dbl, "Chops":bool[]}[]
  T38 = enum32{"invalid app kind", "Development System", "Run Time System", "Student Edition", "Embedded LabVIEW", "Evaluation", "Custom"}
  T39 = enum8{"Enabled", "Disabled", "Disabled and Grayed Out"}
  T40 = enum32{"Invalid", "Standard", "Closed", "Hidden", "Minimized", "Maximized"}
  T41 = cluster{"Font Name:":string, "Size":i16, "Strikeout?":bool, "Italic?":bool, "Underline?":bool, "Outline?":bool, "Shadow?":bool, "Bold?":bool}
  T42 = enum16{"User-specified Font", "Application Font", "System Font", "Dialog Font"}
  T43 = enum16{"None", "Stacked", "Clockwise", "Counterclockwise"}
  T44 = cluster{"horizontal":enum16{"left", "center", "right"}, "vertical":enum16{"top", "center", "bottom"}}
  T45 = enum16{"big-endian, network order", "native, host order", "little-endian"}
  T46 = cluster{"VISA resource name":refnum<visa-resource-name>, "baud rate":u32, "data bits":u16, "parity":u16, "stop bits":u16, "flow control":u16, "termination char\n(0xA = '\\n' = LF)":u8, "timeout (ms)":u32, "End write with termination character?":bool, "End read on termination character?":bool}
  T47 = enum32{"invalid OS target", "Mac OS", "Windows 3.1", "Windows 95/NT", "Solaris 1", "Solaris 2", "HP-UX", "PowerMAX", "Linux", "Irix", "Rhapsody", "BeOS", "AIX", "OSF1", "VxWorks", "PharLap", "Carbon", "RTX", "Windows x64", "Linux x64"}
  T48 = cluster{"load ARR at ioupdate":bool, "ramp enable":bool, "amplitude multiplier enable":bool, "open":bool, "inc/dec step size (14)":bool, "inc/dec step size (15)":bool}
  T49 = cluster{"0=cos, 1=sin":bool, "clear phase accum":bool, "autoclear phase accum":bool, "clear sweep accum":bool, "autoclear sweep accum":bool, "match pipe delays":bool, "DAC power down":bool, "digital power down":bool, "DAC current (8)":bool, "DAC current (9)":bool, "Must be 0":bool, "Open":bool, "Open":bool, "Sweep ramp rate timer":bool, "Sweep enable":bool, "Sweep no-dwell":bool, "Open":bool, "Open":bool, "Open":bool, "Open":bool, "Open":bool, "Open 2":bool, "AFP mod select (22)":bool, "AFP mod select (23)":bool}
  T50 = cluster{"Baud Rate":u32, "Parity":u16, "Data Bits":u16, "Flow Control":u16}
  T51 = cluster{"Bchip":dbl[][], "Status":dbl[], "Temperature":dbl, "Chip":dbl[], "Board":string, "Time Stamp":string}[]
  T52 = cluster{"Core":cluster{"Current VI Reference":refnum<vi>, "Close Panel on Exit?":bool}, "Command History":string[], "Command Names":string[], "Time":u32, "Do Loop Contents":string, "Scan Prefix":path, "Scan Index":u32, "Switch Scan Index":i32, "Switch Scan":bool[][], "Paused":bool, "Paused Queue":string[], "Block Prefix":path, "dac state":cluster{"loaded":bool, "output 1":refnum<k21>, "clock 1":refnum<k21>, "output 2":refnum<k21>, "clock 2":refnum<k21>}, "Block Index":u32, "Idle Timer":u32, "img mcp tcp":refnum<k5>, "TDS5034B Data":cluster{"Y":dbl[], "t0":dbl, "dt":dbl}[], "TDS2014 Data":cluster{"Y":dbl[], "t0":dbl, "dt":dbl}[]}
  T53 = cluster{"Current VI Reference":refnum<vi>, "Close Panel on Exit?":bool}
  T54 = cluster{"Channel":string, "Name":string, "plot":bool}
  T55 = cluster{"Name":string, "DAC":cluster{"Time":dbl, "Voltage":dbl[]}[]}
  T56 = typedef "Rendezvous RefNum" = refnum<k1>
  T57 = cluster{"scan":bool, "Reference":string, "equation":string, "index":i32, "progress":u8, "next":dbl}
  T58 = cluster{"DIO64":cluster{"Task":string, "begin time":dbl, "begin edge":bool, "begin reference":string, "end time":dbl, "end edge":bool, "end reference":string, "Chops":bool[]}[], "DIO64 Tasks":cluster{"Name":string, "DIO64 Line 1":bool[], "DIO64 Line 2":bool[], "DIO64 Line 3":bool[], "DIO64 Line 4":bool[]}[], "Channel Labels":cluster{"Channel":string, "Name":string, "plot":bool}[][], "Current Chops":u16[], "Frames and Rep Rate":cluster{"Frames":i32, "Repetition Rate":dbl}, "Chop Labels":string[]}
  T59 = cluster{"Header":cluster{"Element Names":string[], u8[]}, cluster{"DIO64":cluster{"Task":string, "begin time":dbl, "begin edge":bool, "begin reference":string, "end time":dbl, "end edge":bool, "end reference":string, "Chops":bool[]}[], "DIO64 Tasks":cluster{"Name":string, "DIO64 Line 1":bool[], "DIO64 Line 2":bool[], "DIO64 Line 3":bool[], "DIO64 Line 4":bool[]}[], "Channel Labels":cluster{"Channel":string, "Name":string, "plot":bool}[][], "Current Chops":u16[], "Frames and Rep Rate":cluster{"Frames":i32, "Repetition Rate":dbl}, "Chop Labels":string[]}}
  T60 = cluster{"DAC Schedule":cluster{"Task":string, "Reference":string, "Begin":dbl, "Chops 2":bool[]}[], "DAC Tasks":cluster{"Name":string, "DAC":cluster{"Time":dbl, "Voltage":dbl[]}[]}[], "DAC Kick 2":cluster{"Name":string, "DAC":cluster{"Time":dbl, "Voltage":dbl[]}[]}[]}
  T61 = cluster{"Header":cluster{"Element Names":string[], u8[]}, cluster{"DAC Schedule":cluster{"Task":string, "Reference":string, "Begin":dbl, "Chops 2":bool[]}[], "DAC Tasks":cluster{"Name":string, "DAC":cluster{"Time":dbl, "Voltage":dbl[]}[]}[], "DAC Kick 2":cluster{"Name":string, "DAC":cluster{"Time":dbl, "Voltage":dbl[]}[]}[]}}
  T62 = cluster{"Scan References":cluster{"scan":bool, "Reference":string, "equation":string, "index":i32, "progress":u8, "next":dbl}[], "Scan Variables":cluster{"variable":string, "scan string":string, "randomize":bool, "enable":bool}[]}
  T63 = cluster{"Header":cluster{"Element Names":string[], u8[]}, cluster{"Scan References":cluster{"scan":bool, "Reference":string, "equation":string, "index":i32, "progress":u8, "next":dbl}[], "Scan Variables":cluster{"variable":string, "scan string":string, "randomize":bool, "enable":bool}[]}}
  T64 = cluster{"Jessica":T17, "Bertha":cluster{"wavelength":dbl, "locked":bool, "DIO64":string, "scan start":dbl, "scan end":dbl, "progress":u8, "scan step":dbl, "scan":bool, "setpoint":dbl, "wavelengths":dbl[]}, "Cora":cluster{"wavelength":dbl, "locked":bool, "DIO64":string, "scan start":dbl, "scan end":dbl, "progress":u8, "scan step":dbl, "scan":bool, "setpoint":dbl}, "Stella":cluster{"wavelength":dbl, "locked":bool, "lock tolerance":dbl, "setpoint":dbl, "scan start":dbl, "scan end":dbl, "progress":u8, "scan step":dbl, "scan":bool, "AI Channel":tag}, "Toptica":cluster{"wavelength":dbl, "locked":bool, "scan start":dbl, "scan end":dbl, "progress":u8, "scan step":dbl, "scan":bool, "AI Channel":tag}, "TiSapph":cluster{"wavelength":dbl, "scan start":dbl, "scan end":dbl, "progress":u8, "scan step":dbl, "scan":bool, "setpoint":dbl, "wavelengths":dbl[], "Channel":tag, "wavelength 2":dbl}}
  T65 = cluster{"Header":cluster{"Element Names":string[], u8[]}, cluster{"Jessica":T17, "Bertha":cluster{"wavelength":dbl, "locked":bool, "DIO64":string, "scan start":dbl, "scan end":dbl, "progress":u8, "scan step":dbl, "scan":bool, "setpoint":dbl, "wavelengths":dbl[]}, "Cora":cluster{"wavelength":dbl, "locked":bool, "DIO64":string, "scan start":dbl, "scan end":dbl, "progress":u8, "scan step":dbl, "scan":bool, "setpoint":dbl}, "Stella":cluster{"wavelength":dbl, "locked":bool, "lock tolerance":dbl, "setpoint":dbl, "scan start":dbl, "scan end":dbl, "progress":u8, "scan step":dbl, "scan":bool, "AI Channel":tag}, "Toptica":cluster{"wavelength":dbl, "locked":bool, "scan start":dbl, "scan end":dbl, "progress":u8, "scan step":dbl, "scan":bool, "AI Channel":tag}, "TiSapph":cluster{"wavelength":dbl, "scan start":dbl, "scan end":dbl, "progress":u8, "scan step":dbl, "scan":bool, "setpoint":dbl, "wavelengths":dbl[], "Channel":tag, "wavelength 2":dbl}}}
  T66 = cluster{"DDS":cluster{"address":refnum<visa-resource-name>, "channel 1":dbl, "channel 2":dbl, "channel 3":dbl, "channel 4":dbl, "clock":dbl, "pll multiplier":u8, "vco gain":bool, "detected":bool, "channel 1 endramp":dbl, "channel 2 endramp":dbl, "channel 3 endramp":dbl, "channel 4 endramp":dbl, "frequency ramp":bool}}
  T67 = cluster{"Header":cluster{"Element Names":string[], u8[]}, cluster{"DDS":cluster{"address":refnum<visa-resource-name>, "channel 1":dbl, "channel 2":dbl, "channel 3":dbl, "channel 4":dbl, "clock":dbl, "pll multiplier":u8, "vco gain":bool, "detected":bool, "channel 1 endramp":dbl, "channel 2 endramp":dbl, "channel 3 endramp":dbl, "channel 4 endramp":dbl, "frequency ramp":bool}}}
  T68 = cluster{"Trap DDS":cluster{"channels":cluster{"Frequency":dbl, "Phase":dbl, "Amplitude":dbl}[], "usb 1":refnum<visa-resource-name>, "usb 2":refnum<visa-resource-name>, "clock":dbl, "pll multiplier":u8, "ioupdate":bool, "detected":bool, "ramp":cluster{"start":dbl, "end":dbl, "ramp time":u8, "edge":bool}[], "232":refnum<visa-resource-name>, "load ARR":bool, "ramp enable":bool, "ramp time":u8, "Global\nScale Factor":dbl}}
  T69 = cluster{"Header":cluster{"Element Names":string[], u8[]}, cluster{"Trap DDS":cluster{"channels":cluster{"Frequency":dbl, "Phase":dbl, "Amplitude":dbl}[], "usb 1":refnum<visa-resource-name>, "usb 2":refnum<visa-resource-name>, "clock":dbl, "pll multiplier":u8, "ioupdate":bool, "detected":bool, "ramp":cluster{"start":dbl, "end":dbl, "ramp time":u8, "edge":bool}[], "232":refnum<visa-resource-name>, "load ARR":bool, "ramp enable":bool, "ramp time":u8, "Global\nScale Factor":dbl}}}
  T70 = cluster{"Measure Commands":string, "Test Commands":string, "Functions":cluster{"Name":string, "Body":string}[], "Chops":cluster{"Chops":u16[]}[]}
  T71 = cluster{"Header":cluster{"Element Names":string[], u8[]}, cluster{"Measure Commands":string, "Test Commands":string, "Functions":cluster{"Name":string, "Body":string}[], "Chops":cluster{"Chops":u16[]}[]}}
  T72 = cluster{"date string":string, "time string":string}
  T73 = cluster{"Header":cluster{"Element Names":string[], u8[]}, cluster{"date string":string, "time string":string}}
  T74 = cluster{"Machine State":cluster{"Brot":bool, "Doublet":bool, "Rotation":bool, "Depletion phase":bool, "Depletion pol":bool}, "Switch Settings":cluster{"Brot":cluster{"in":dbl, "out":dbl}, "Doublet":cluster{"upper":dbl, "lower":dbl, "DurationUpper":dbl, "DurationLower":dbl, "Upper T":dbl, "Lower T":dbl}, "Rotation":cluster{"Down":cluster{"Frequency":dbl, "Phase":dbl, "Amplitude":dbl}[], "Up":cluster{"Frequency":dbl, "Phase":dbl, "Amplitude":dbl}[]}, "Depletion phase":cluster{"0 phase":dbl, "pi phase":dbl}}}
  T75 = cluster{"Header":cluster{"Element Names":string[], u8[]}, cluster{"Machine State":cluster{"Brot":bool, "Doublet":bool, "Rotation":bool, "Depletion phase":bool, "Depletion pol":bool}, "Switch Settings":cluster{"Brot":cluster{"in":dbl, "out":dbl}, "Doublet":cluster{"upper":dbl, "lower":dbl, "DurationUpper":dbl, "DurationLower":dbl, "Upper T":dbl, "Lower T":dbl}, "Rotation":cluster{"Down":cluster{"Frequency":dbl, "Phase":dbl, "Amplitude":dbl}[], "Up":cluster{"Frequency":dbl, "Phase":dbl, "Amplitude":dbl}[]}, "Depletion phase":cluster{"0 phase":dbl, "pi phase":dbl}}}}
